vi "my_spectrogram_display.vi"(4 "Modulation info":T1={"Fs full"=0.0, "Fs high"=0.0, "Fs low"=0.0, "Read size"=0, "FFT size low"=5000, "df low"=5000.0, "High carriers"=[], "Low carriers"=[], "Hi channels at low"=[7]} {"Hi channels at low" min=0 step=1; "Low carriers" format="%#_6p"; "High carriers" format="%#_6p"}, 6 "time-freq sample info":cluster{"time steps":i32, "frequency bins":i32}, 8 "Map selector":T2(ring)=enum."rainbow", 9 "IntensityGraph in":refnum<vi>, 10 "dB On":bool=TRUE, 11 "STFT {X}":cdb[][](array[numeric]) format="%#_4p") -> (2 "STFT Spectrogram":dbl[][](graph))   [LabVIEW 2014]
uses:
  modulation_info.ctl
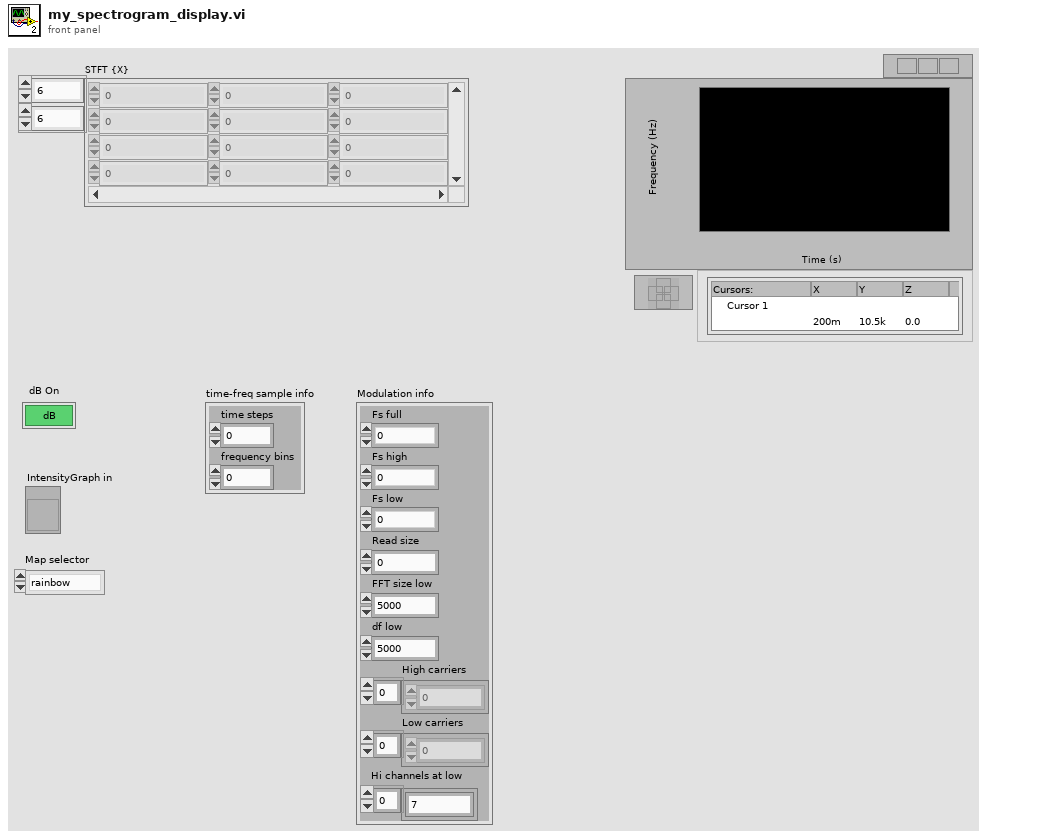
[diagram p1: front panel]
types:
  T1 = typedef "modulation_info.ctl" = cluster{"Fs full":dbl, "Fs high":dbl, "Fs low":dbl, "Read size":i32, "FFT size low":i32, "df low":dbl, "High carriers":dbl[], "Low carriers":dbl[], "Hi channels at low":i32[]}
  T2 = enum16{"fire", "rainbow", "grey", "inverse grey", "ice", "original"}
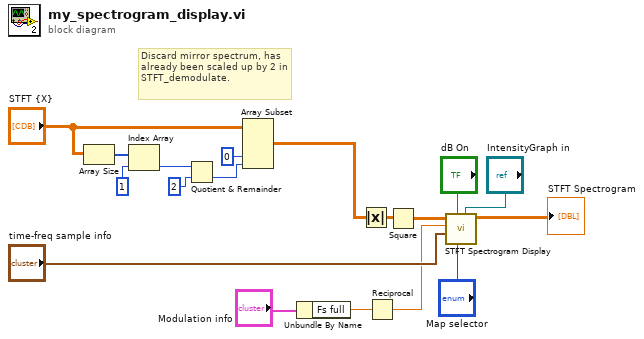
[diagram p0: block diagram]
diagram:
  # "Discard mirror spectrum, has already been scaled up by 2 in STFT_demodulate."
  n1 = Array Size(array="STFT {X}") -> (size(s)=w7:i32[])
  n2 = Index Array(array=w7, index=1) -> (element=w5:i32)
  n3 = Quotient & Remainder(x=w5, y=2) -> (floor(x/y)=w10:i32)  [unwired: 1 out]
  n4 = Array Subset(array="STFT {X}", index (col)=0 ("index"), length (col)=w10) -> (w2:cdb[][])  [unwired: 2 in]
  n5 = Unbundle By Name("Modulation info") -> ("Fs full"=w8:dbl)
  n6 = Absolute Value(x=w2) -> (abs(x)=w17:dbl[][])
  n7 = Reciprocal(x=w8) -> (1/x=w1:dbl)
  n8 = Square(x=w17) -> (x^2=w18:dbl[][])
  n9 = call "STFT Spectrogram Display.vi"("Intensity Graph"="IntensityGraph in", "map selector"="Map selector", "dB On"="dB On", "time-freq sampling info"="time-freq sample info", "dt"=w1, "STFT Spectrogram In"=w18) -> ("STFT Spectrogram Out"=→"STFT Spectrogram":dbl[][])  [unwired: 4 in, 1 out]
